vi "Abscissas Generator.vi"(10 "upper limit":dbl, 11 "lower limit":dbl) -> (2 "4 points":dbl[](array[numeric]), 3 "7 points":dbl[](array[numeric]))   [LabVIEW 2017, in "NI_AALPro.lvlib"]
uses:
  NI_AALPro.lvlib
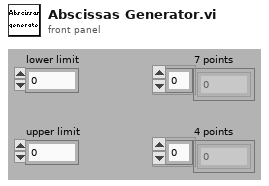
[diagram p1: front panel]
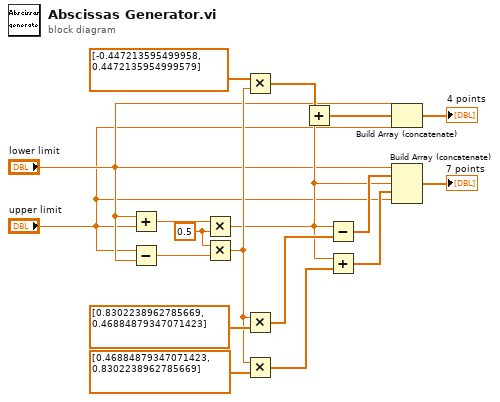
[diagram p0: block diagram]
diagram:
  w1 = 0.5 ("y")
  n1 = Add(x="lower limit", y="upper limit") -> (x+y=w14:dbl)
  n2 = Subtract(x="upper limit", y="lower limit") -> (x-y=w13:dbl)
  n3 = Multiply(x=w14, y=w1) -> (x*y=w8:dbl)
  n4 = Multiply(x=w1, y=w13) -> (x*y=w10:dbl)
  n5 = Multiply(x=dbl[] [-0.447213595499958, 0.4472135954999579] ("appended array"), y=w10) -> (x*y=w9:dbl[])
  n6 = Multiply(x=w10, y=dbl[] [0.8302238962785669, 0.46884879347071423] ("appended array")) -> (x*y=w18:dbl[])
  n7 = Multiply(x=w10, y=dbl[] [0.46884879347071423, 0.8302238962785669] ("appended array")) -> (x*y=w17:dbl[])
  n8 = Add(x=w9, y=w8) -> (x+y=w7:dbl[])
  n9 = Subtract(x=w8, y=w18) -> (x-y=w16:dbl[])
  n10 = Add(x=w8, y=w17) -> (x+y=w15:dbl[])
  n11 = Build Array (concatenate)("lower limit", w7, "upper limit") -> (→"4 points":dbl[])
  n12 = Build Array (concatenate)("lower limit", w16, w8, w15, "upper limit") -> (→"7 points":dbl[])
